vi "J1939 - Workspace Control.vi"() -> ()   [LabVIEW 2019, in "J1939 Workspace Object.lvlib"]
doc: "Sample numeric display item."
uses:
  J1939 Workspace Object.lvlib
  <vilib>/NI VeriStand/Display Template Support/DisplayTemplateSupport.llb/cluster_Screen Item Settings.ctl
  <vilib>/NI VeriStand/Display Template Support/DisplayTemplateSupport.llb/cluster_Graph Scale Settings.ctl
  <vilib>/NI VeriStand/Display Template Support/DisplayTemplateSupport.llb/cluster_Graph Plot Settings.ctl
  NationalInstruments.VeriStand.SystemStorage
  Workspace Shared/Types/UI.StateVariables.ctl
  <vilib>/NI VeriStand/Display Template Support/DisplayTemplateSupport.llb/enum_Display Template Handler Minimal To Widget Msg.ctl
  <vilib>/NI VeriStand/Execution/Workspace/SystemStateRegEventRef.ctl
  <vilib>/NI VeriStand/Execution/Workspace/Target State Info.ctl
  <vilib>/NI VeriStand/Execution/Workspace/Target State.ctl
  Shared/Types/Private Data.ctl
  <vilib>/NI/STM/TCP/TCP Connection Info.ctl
  <vilib>/NI/STM/SubVIs/MetaDataElement.ctl
  Shared/Types/Error Cluster.ctl
  Shared/Types/Error Types.ctl
  <vilib>/NI VeriStand/Display Template Support/DisplayTemplateSupport.llb/enum_Display Template Handler Minimal To Workspace.ctl
  <vilib>/NI VeriStand/Execution/Workspace/WorkspaceAPI.ctl
  <vilib>/NI VeriStand/Execution/Workspace/SystemStateEventRef.ctl
  Workspace Shared/Types/UI.Refs.ctl
  <vilib>/Utility/miscctls.llb/LVStringsAndValuesArrayTypeDef_U8.ctl
  Shared/J1939 Utilities/SubVIs/Convert CAN Arb ID to J1939 ID.vi
  <vilib>/NI VeriStand/Display Template Support/DisplayTemplateSupport.llb/sub_Display Template Handler Custom.vi
  Shared/J1939 Addon Shared.lvlib
  <vilib>/NI/STM/NI STM.lvlib
  Workspace Shared/J1939 Workspace Shared.lvlib
  <vilib>/NI VeriStand/Execution/Workspace/NI_VS Workspace ExecutionAPI.lvlib
  Shared/J1939 Utilities/J1939 Utilities.lvlib
  NationalInstruments.VeriStand.ClientAPI
panel:
  in  "Tab Control":enum32{"DTCs", "Custom RQST", "RAW FRAME"}(tab)
  in  "Refresh Continuous":bool
  in  "Clear DTC":bool
  in  "Refresh DTCs":bool
  in  "DTCs":i32(listbox)
  in  "Addresses":string(tree)
  in  "Refresh Addresses":bool
  out "Response":string
  in  "Request":bool
  in  "PGN":u32 format="%.0x"
  in  "DA":u8(ring)
  in  "Clear Array":bool
  in  "RAW":bool
  out "Priority":u8 format="%02x"
  out "SA":u8 format="%02x"
  out "PGN":u32 format="%06x"
  in  "Identifier":u32 format="%08x"
  in  "Data":u8[](array[numeric])=[0, 0, 0, 0, 0, 0, 0, 0] format="%.0x"
  in  "Errors":bool
  out "Device":string
  in  "NIVS.Workspace Event":refnum<event-registration>
  in  "NIVS.Gateway IP Address":string
  in  "NIVS.System Definition Root":refnum<k24>
  in  "Item.Data":T1
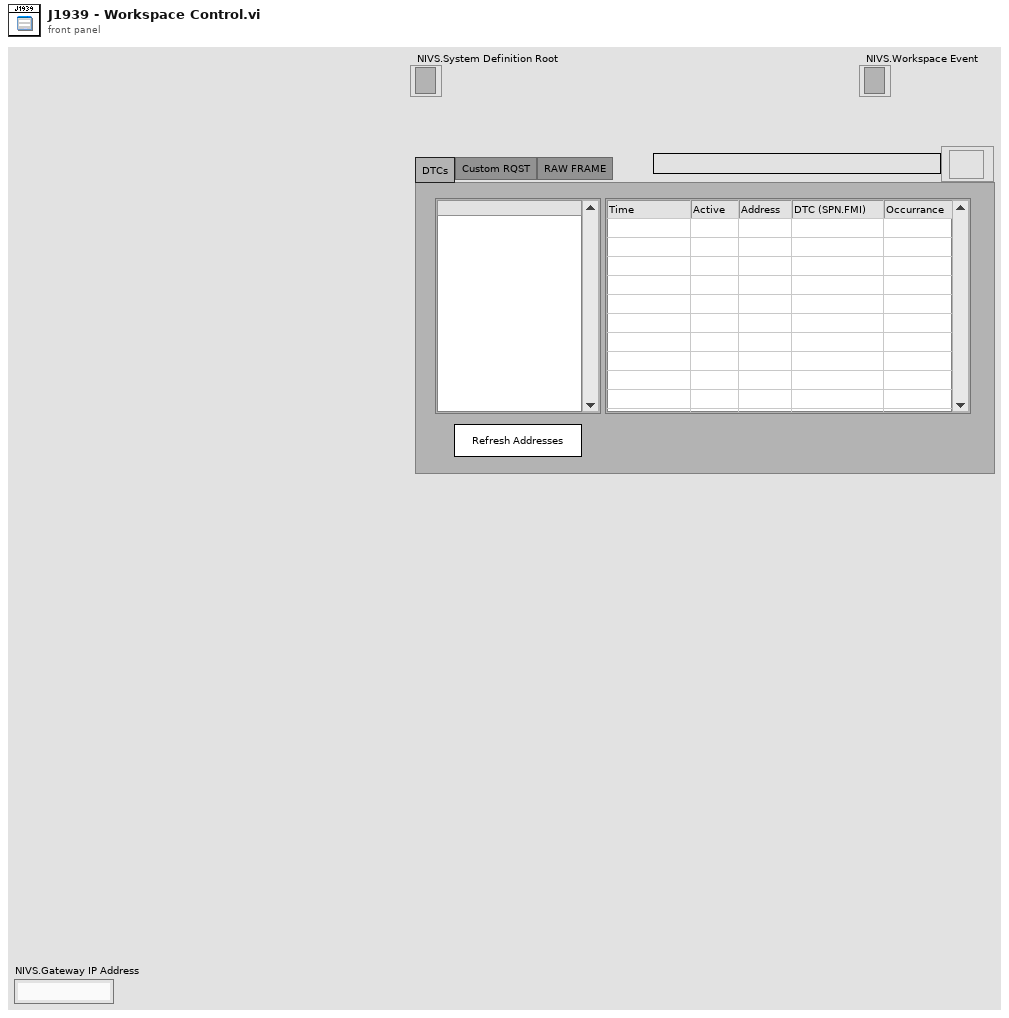
[diagram p1: front panel]
types:
  T1 = typedef "cluster_Screen Item Settings.ctl" = cluster{"Template VI":string, "Position X":i32, "Position Y":i32, "Custom":string, "Show Title Bar":bool, "ID":i32, "Always On Top":bool, "Allow Resize":bool, "Allow Minimize":bool, "Allow Close":bool, "Size to Screen":bool, "Screen.ID":i32, "State":enum16{"Normal", "New"}, "Title":string, "Window Bounds":cluster{"[0]":i16, "[1]":i16, "[2]":i16, "[3]":i16}, "Channel Ref":u64, "Unit":string, "Default Units?":bool, "Flash Limit?":bool, "Color 1":u32, "Color 2":u32, "Color 3":u32, "Color 4":u32, "Bck Color":u32, "Fore Color":u32, "Limit 1":dbl, "Limit 2":dbl, "Limit 3":dbl, "Limit 4":dbl, "Limit Mode 1":i32, "Limit Mode 2":i32, "Limit Mode 3":i32, "Limit Mode 4":i32, "Scale Precision":i32, "Scale Min":dbl, "Scale Max":dbl, "Format":i32, "Precision":i32, "Background Type":i32, "IDs":i32[], "Units":string[], "Labels":string[], "Scale Factor":dbl, "Scale Offset":dbl, "YScale Index":u32[], "XScale":T2, "YScales":T2[], "Plots":T3[], "Update Period":dbl, "History Length":dbl, "My.Ref":refnum<vi>, "Is Control?":bool, "Channel Paths":string[], "Custom Data":variant}
  T2 = typedef "cluster_Graph Scale Settings.ctl" = cluster{"Format":u8, "Precision":u8, "Fit":u8, "Label":string, "Use Default Label":bool, "Label Visible":bool, "Min":dbl, "Max":dbl}
  T3 = typedef "cluster_Graph Plot Settings.ctl" = cluster{"Bar Style":u8, "Fill To":i16, "Fill/PtColor":u32, "Line Style":u8, "Line Width":u8, "Color":u32, "Interp":u8, "Point Style":u8}
  T4 = typedef "J1939 Workspace Shared.lvlib/UI.StateVariables.ctl" = cluster{"NIVS.Gateway IP Address":string, "LaunchConfig.Ref":refnum<user-event>, "Events.Refs":cluster{"LaunchConfig":refnum<event-registration>, "SystemChange":T5, "NIVS.Workspace":refnum<event-registration>}, "State":T6, "TCP.Refs":T7, "Addresses.LUT":variant, "Errors.Q":refnum<queue>, "NIVS.SysDefRoot":refnum<k24>, "State.Notifier":refnum<user-event>, "NIVS.Workspace":T9, "DTCs.Refresh":bool, "NIVS.State.Refs":T10, "UI.Refs":T11, "Addon.Connected":bool, "DTCs.Timer":u32, "Mode.Tool?":bool}
  T5 = typedef "NI_VS Workspace ExecutionAPI.lvlib/SystemStateRegEventRef.ctl" = refnum<event-registration>
  T6 = typedef "J1939 Addon Shared.lvlib/Private Data.ctl" = cluster{"PGN":u32, "DA":u8, "CD Path":string, "CD IP":string}
  T7 = typedef "NI STM.lvlib/TCP Connection Info.ctl" = cluster{"connection ID":refnum<k5>, "meta data":T8[]}
  T8 = typedef "NI STM.lvlib/MetaDataElement.ctl" = string
  T9 = typedef "NI_VS Workspace ExecutionAPI.lvlib/WorkspaceAPI.ctl" = refnum<k24>
  T10 = typedef "NI_VS Workspace ExecutionAPI.lvlib/SystemStateEventRef.ctl" = cluster{"CustDatRef":refnum<user-event>, "EvtRef":refnum<k27>, "Target State User Event":refnum<user-event>}
  T11 = typedef "J1939 Workspace Shared.lvlib/UI.Refs.ctl" = cluster{"ParentVI":refnum<vi>, "DTCs":refnum<vi>, "Addresses":refnum<vi>, "Device":refnum<vi>, "Data":refnum<vi>, "Identifier":refnum<vi>, "PGN":refnum<vi>, "DA":refnum<vi>, "Refresh Continuous":refnum<vi>, "Errors":refnum<vi>, "Refresh Addresses":refnum<vi>, "Refresh DTCs":refnum<vi>, "Clear DTC":refnum<vi>, "Request":refnum<vi>, "Clear Array":refnum<vi>, "RAW":refnum<vi>, "SA":refnum<vi>, "PGN Ind":refnum<vi>, "Priority":refnum<vi>, "Response":refnum<vi>}
  T12 = typedef "enum_Display Template Handler Minimal To Workspace.ctl" = cluster{"Operation":enum16{"SetCustomData", "DeleteItem"}, "Data":variant}
  T13 = typedef "enum_Display Template Handler Minimal To Widget Msg.ctl" = enum16{"Stop", "LaunchConfigDialog"}
  T14 = enum8{"Enabled", "Disabled", "Disabled and Grayed Out"}
  T15 = typedef "LVStringsAndValuesArrayTypeDef_U8.ctl" = cluster{"String":string, "Value":u8}[]
  T16 = cluster{"LaunchConfig":refnum<event-registration>, "SystemChange":T5, "NIVS.Workspace":refnum<event-registration>}
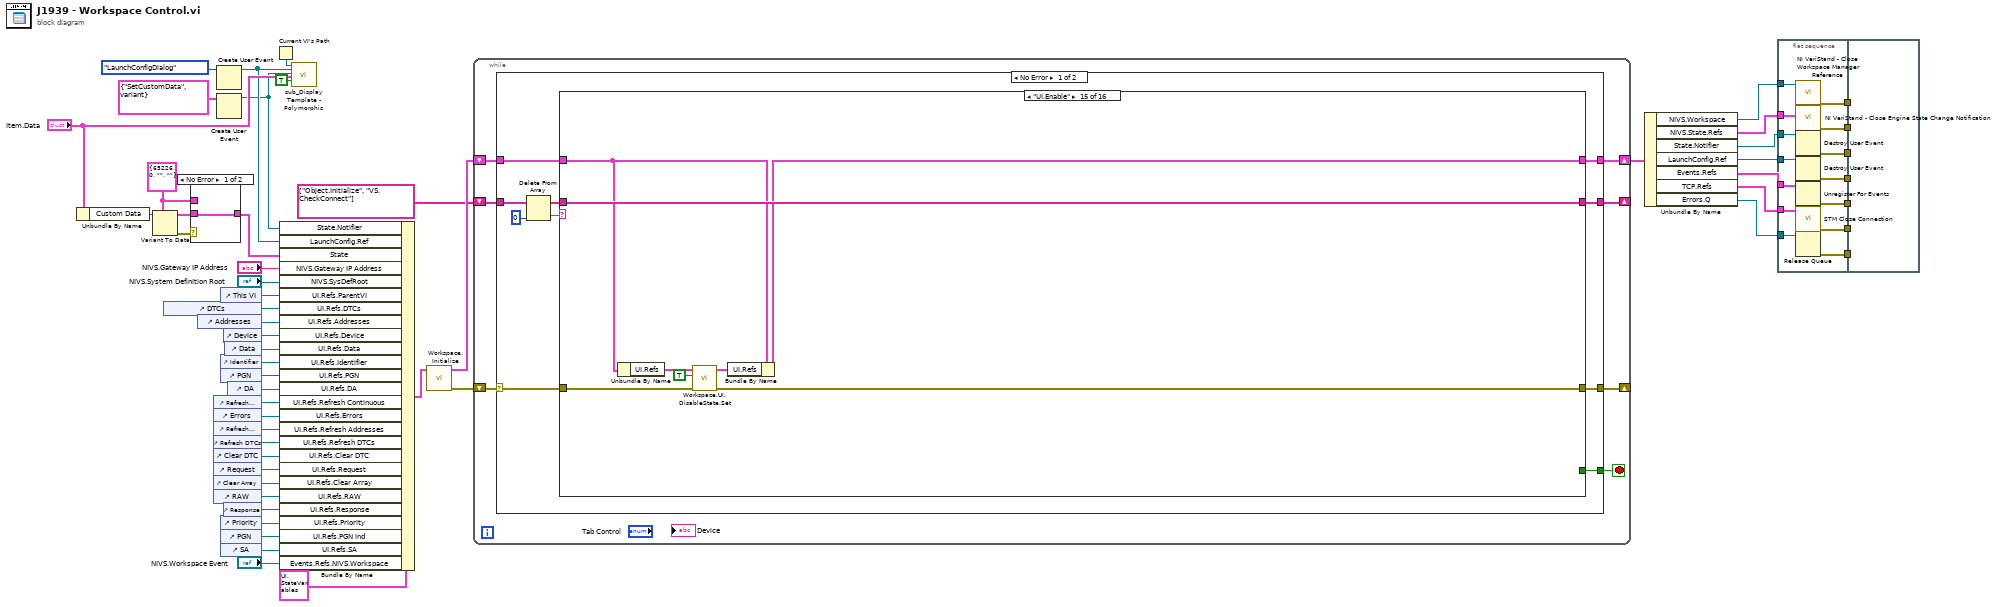
[diagram p0: block diagram]
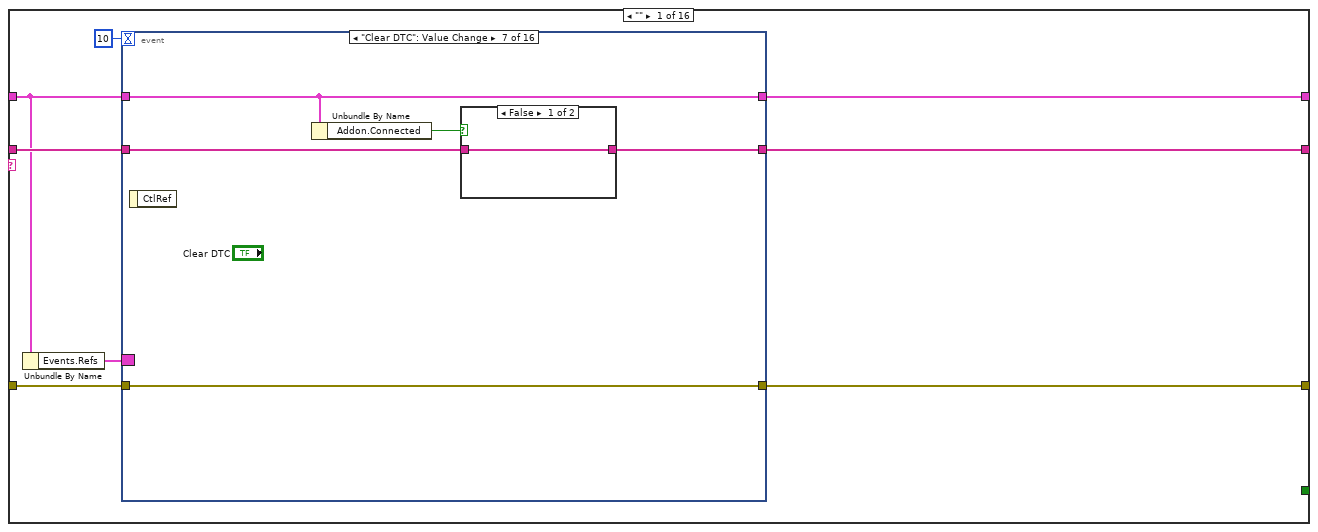
[diagram p2: hidden frame]
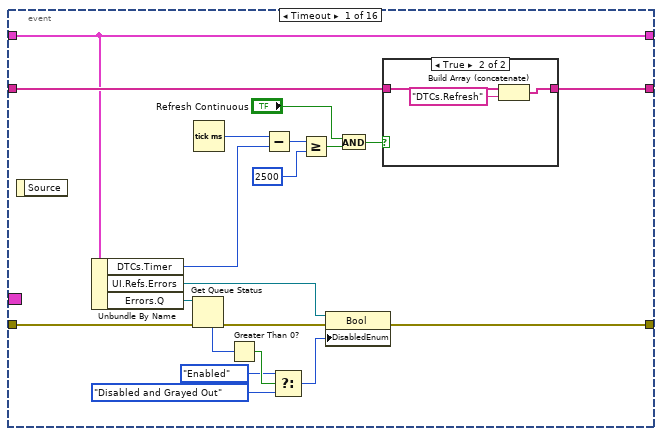
[diagram p3: hidden frame]
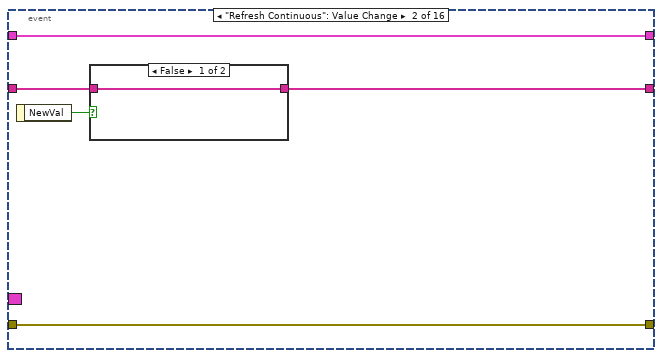
[diagram p5: hidden frame]
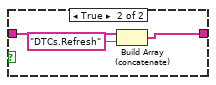
[diagram p6: hidden frame]
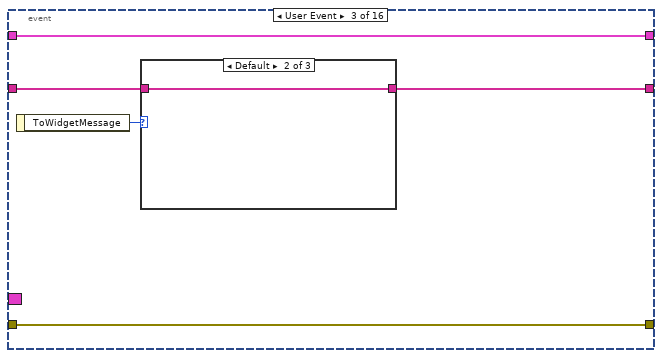
[diagram p7: hidden frame]
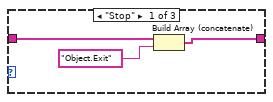
[diagram p8: hidden frame]
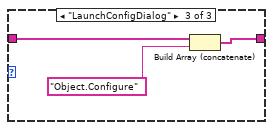
[diagram p9: hidden frame]
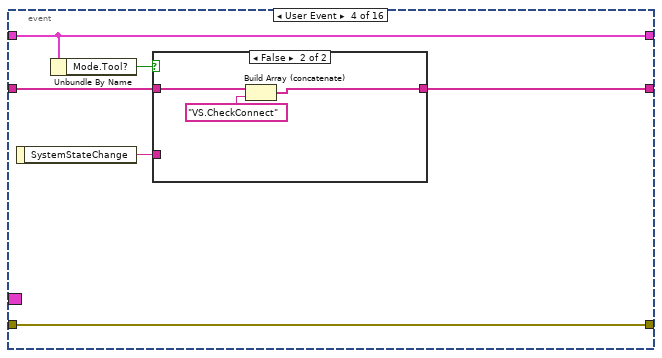
[diagram p10: hidden frame]
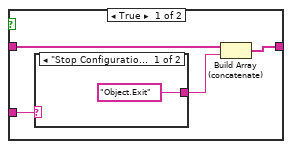
[diagram p11: hidden frame]
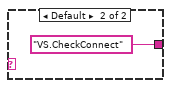
[diagram p12: hidden frame]
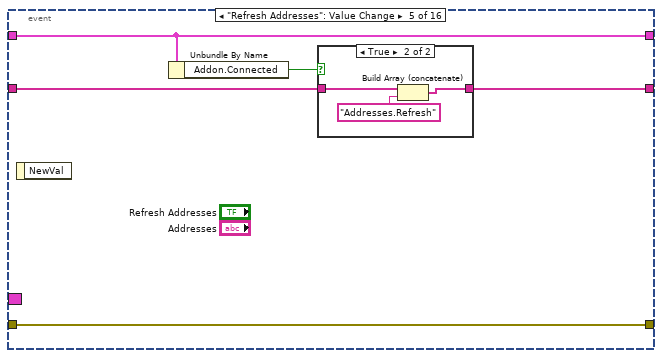
[diagram p13: hidden frame]
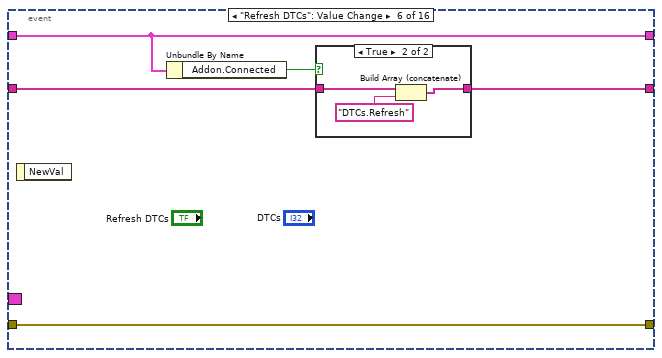
[diagram p15: hidden frame]
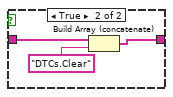
[diagram p17: hidden frame]
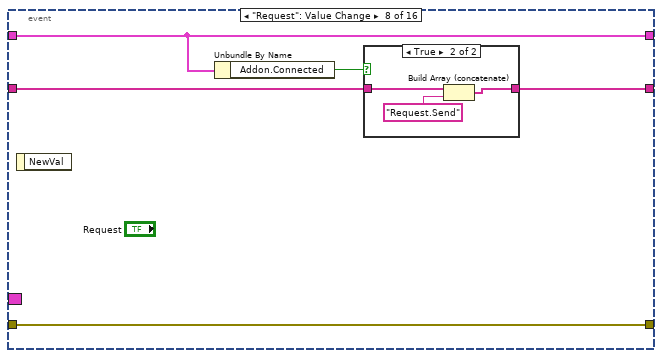
[diagram p18: hidden frame]
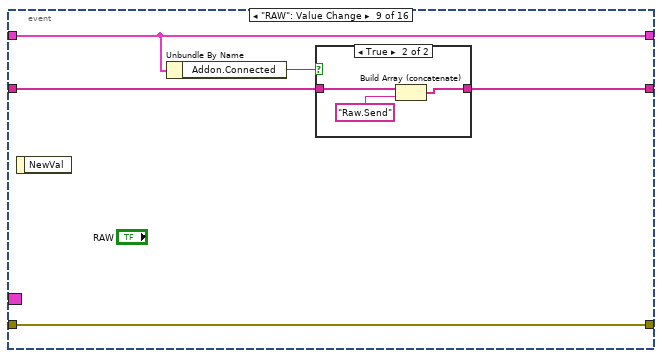
[diagram p20: hidden frame]
diagram:
  w51 = T6 {"PGN"=65226, "DA"=0, "CD Path"="", "CD IP"=""} ("Cluster")
  n1 = Unbundle By Name("Item.Data") -> ("Custom Data"=w48:variant)
  n2 = Variant To Data(type=w51, Variant=w48) -> (data=w50:T6, error out=w49:errorcluster)  [unwired: 1 in]
  n3 = control-ref of="DTCs"() -> (w35:refnum<vi>)
  n4 = case shown="No Error" w49 {
    tunnel: w50 -> [w56 _]
    tunnel: [w56 w57] -> w7
    tunnel: w51 -> [_ w57]
    frame No Error {
    }
    frame Error {
    }
  }
  n5 = control-ref of="Addresses"() -> (w34:refnum<vi>)
  n6 = control-ref of="Refresh Continuous"() -> (w28:refnum<vi>)
  n7 = control-ref of="Errors"() -> (w27:refnum<vi>)
  n8 = control-ref of="Refresh Addresses"() -> (w26:refnum<vi>)
  n9 = control-ref of="Refresh DTCs"() -> (w25:refnum<vi>)
  n10 = control-ref of="Clear DTC"() -> (w24:refnum<vi>)
  n11 = control-ref of="Request"() -> (w23:refnum<vi>)
  n12 = control-ref of="Clear Array"() -> (w22:refnum<vi>)
  n13 = control-ref of="RAW"() -> (w21:refnum<vi>)
  n14 = Create User Event(user event datatype=enum_Display_Template_Handler_Minimal_To_Widget_Msg."LaunchConfigDialog" ("ToWidgetMessage")) -> (user event=w6:refnum<user-event>)  [unwired: 1 in, 1 out]
  n15 = Create User Event(user event datatype=T12 {"Operation"=enum."SetCustomData", "Data"=variant} ("Data")) -> (user event=w5:refnum<user-event>)  [unwired: 1 in, 1 out]
  n16 = control-ref of="This VI"() -> (w36:refnum<vi>)
  n17 = control-ref of="Identifier"() -> (w31:refnum<vi>)
  n18 = control-ref of="PGN"() -> (w30:refnum<vi>)
  n19 = control-ref of="Priority"() -> (w2:refnum<vi>)
  n20 = control-ref of="PGN"() -> (w3:refnum<vi>)
  n21 = control-ref of="SA"() -> (w4:refnum<vi>)
  n22 = control-ref of="Device"() -> (w33:refnum<vi>)
  n23 = control-ref of="Response"() -> (w1:refnum<vi>)
  n24 = control-ref of="Data"() -> (w32:refnum<vi>)
  n25 = control-ref of="DA"() -> (w29:refnum<vi>)
  n26 = Current VI's Path() -> (path=w53:path)
  n27 = Bundle By Name(cluster=T4 {"NIVS.Gateway IP Address"="", "LaunchConfig.Ref"=refnum, "Events.Refs"={"LaunchConfig"=refnum, "SystemChange"=refnum, "NIVS.Workspace"=refnum}, "State"={"PGN"=0, "DA"=0, "CD Path"="", "CD IP"=""}, "TCP.Refs"={"connection ID"=refnum, "meta data"=[]}, "Addresses.LUT"=variant, "Errors.Q"=refnum, "NIVS.SysDefRoot"=refnum, "State.Notifier"=refnum, "NIVS.Workspace"=refnum, "DTCs.Refresh"=FALSE, "NIVS.State.Refs"={"CustDatRef"=refnum, "EvtRef"=refnum, "Target State User Event"=refnum}, "UI.Refs"={"ParentVI"=refnum, "DTCs"=refnum, "Addresses"=refnum, "Device"=refnum, "Data"=refnum, "Identifier"=refnum, "PGN"=refnum, "DA"=refnum, "Refresh Continuous"=refnum, "Errors"=refnum, "Refresh Addresses"=refnum, "Refresh DTCs"=refnum, "Clear DTC"=refnum, "Request"=refnum, "Clear Array"=refnum, "RAW"=refnum, "SA"=refnum, "PGN Ind"=refnum, "Priority"=refnum, "Response"=refnum}, "Addon.Connected"=FALSE, "DTCs.Timer"=0, "Mode.Tool?"=FALSE}, "State.Notifier"=w5, "LaunchConfig.Ref"=w6, "State"=w7, "NIVS.Gateway IP Address"="NIVS.Gateway IP Address", "NIVS.SysDefRoot"="NIVS.System Definition Root", "UI.Refs.ParentVI"=w36, "UI.Refs.DTCs"=w35, "UI.Refs.Addresses"=w34, "UI.Refs.Device"=w33, "UI.Refs.Data"=w32, "UI.Refs.Identifier"=w31, "UI.Refs.PGN"=w30, "UI.Refs.DA"=w29, "UI.Refs.Refresh Continuous"=w28, "UI.Refs.Errors"=w27, "UI.Refs.Refresh Addresses"=w26, "UI.Refs.Refresh DTCs"=w25, "UI.Refs.Clear DTC"=w24, "UI.Refs.Request"=w23, "UI.Refs.Clear Array"=w22, "UI.Refs.RAW"=w21, "UI.Refs.Response"=w1, "UI.Refs.Priority"=w2, "UI.Refs.PGN Ind"=w3, "UI.Refs.SA"=w4, "Events.Refs.NIVS.Workspace"="NIVS.Workspace Event") -> (w38:T4)
  n28 = call-poly <vilib>:"sub_Display Template - Polymorphic.vi"("Parent.Path"=w53, "ToWidgetEvent"=w6, "ToWorkspace"=w5, "Item.Data"="Item.Data", "Resizable"=TRUE) -> ()  [unwired: 1 in, 14 out]
  n29 = call "Workspace.Initialize.vi"("State"=w38) -> ("error out"=w37:errorcluster, "State"=w20:T4)  [unwired: 9 in]
  n30 = while {
    shift-right: [w62] -> _
    shift-left: w37 -> [w63]
    shift-right: [w58] -> w18
    shift-left: w20 -> [w61]
    shift-right: [w59] -> _
    shift-left: string[] ["Object.Initialize", "VS.CheckConnect"] -> [w60]
    stop <- w64 stop-if-true
    n31 = case shown="No Error" w63 {
      selector: w63 -> [w65 w473]
      tunnel: [w74 FALSE] -> w64
      tunnel: [w66 w471] -> w62
      tunnel: w61 -> [w73 w468]
      tunnel: w60 -> [w71 w469]
      tunnel: [w68 w469] -> w59
      tunnel: [w67 w468] -> w58
      frame No Error {
        n32 = Delete From Array(array=w71, index=0) -> (deleted portion=w70:string, array with subset deleted=w69:string[])  [unwired: 1 in]
        n33 = case shown="\"UI.Enable\"" w70 {
          selector: w70 -> [_ _ _ _ _ _ _ _ _ _ _ _ _ _ _ w463]
          tunnel: [_ _ _ _ _ _ _ _ TRUE _ _ _ _ _ _ _] -> w74
          tunnel: w73 -> [w76 w239 w248 w265 w318 w323 w357 w385 w388 w393 w417 w425 w437 w449 w454 w466]
          tunnel: w69 -> [w80 w246 w258 w274 w319 w321 w363 w381 w389 w391 w418 w426 w433 w451 w461 w467]
          tunnel: [w81 w246 w258 w274 w319 w320 w362 w381 w389 w390 w418 w426 w433 w451 w461 w467] -> w68
          tunnel: [w79 w236 w247 w275 w318 w322 w356 w384 w388 w394 w417 w424 w434 w450 w455 w466] -> w67
          tunnel: [w78 w235 w257 w260 w295 w326 w359 w380 w387 w402 w413 w419 w432 w452 w456 w465] -> w66
          tunnel: w65 -> [w77 w235 w257 w261 w292 w327 w358 w380 w387 w403 w412 w419 w432 w453 w457 w465]
          frame "" {
            n34 = Unbundle By Name(w76) -> ("Events.Refs"=w75:T16)
            n35 = event shown="[6] \"Clear DTC\": Value Change" {
              selector: w75 -> [_ _ _ _ _ _ _ _ _ _ _ _ _ _ _ _]
              dyn-events: _ -> [_ _ _ _ _ _ _ _ _ _ _ _ _ _ _ _]
              timeout: 10 -> [_ _ _ _ _ _ _ _ _ _ _ _ _ _ _ _]
              tunnel: w76 -> [w91 w110 w120 w129 w146 w154 w161 w172 w181 w190 w199 w203 w210 w220 w225 w234]
              tunnel: [w92 w108 w116 w132 w144 w152 w162 w170 w179 w188 w198 w204 w212 w216 w222 w231] -> w81
              tunnel: w80 -> [w93 w109 w117 w133 w145 w153 w163 w171 w180 w189 w201 w204 w212 w217 w223 w232]
              tunnel: [w91 w110 w120 w129 w146 w154 w161 w172 w181 w190 w199 w203 w210 w220 w225 w234] -> w79
              tunnel: [w85 w111 w119 w130 w147 w156 w165 w174 w183 w192 w200 w202 w211 w219 w224 w233] -> w78
              tunnel: w77 -> [w87 w111 w119 w130 w147 w156 w165 w174 w183 w192 w200 w202 w211 w219 w224 w233]
              event Timeout {
                n36 = event-data() -> ()  [unwired: 2 out]
                n37 = Unbundle By Name(w91) -> ("DTCs.Timer"=w84:u32, "UI.Refs.Errors"=w89:refnum<vi>, "Errors.Q"=w90:refnum<queue>)
                n38 = Get Queue Status(queue=w90, error in (no error)=w87) -> (error out=w88:errorcluster, # elements in queue=w102:i32)  [unwired: 1 in, 6 out]
                n39 = Tick Count (ms)() -> (millisecond timer value=w96:u32)
                n40 = Greater Than 0?(x=w102) -> (x > 0?=w101:bool)
                n41 = Subtract(x=w96, y=w84) -> (x-y=w98:u32)
                n42 = Select(t=T14."Enabled" ("Disabled"), s=w101, f=T14."Disabled and Grayed Out") -> (s? t:f=w86:T14)
                n43 = Greater Or Equal?(x=w98, y=u32 2500) -> (x >= y?=w83:bool)
                n44 = property class="Bool"(reference=w89, error in=w88, "DisabledEnum"=w86) -> (error out=w85:errorcluster)  [unwired: 1 out]
                n45 = And(x="Refresh Continuous", y=w83) -> (x .and. y?=w94:bool)
                n46 = case shown="True" w94 {
                  tunnel: w93 -> [w103 w105]
                  tunnel: [w103 w104] -> w92
                  frame False {
                  }
                  frame True {
                    n47 = Build Array (concatenate)(w105, "DTCs.Refresh" ("NewVal")) -> (w104:string[])
                  }
                }
              }
              event "Refresh Continuous": Value Change {
                n48 = event-data() -> ("NewVal"=w107:bool)  [unwired: 1 out]
                n49 = case shown="False" w107 {
                  tunnel: w109 -> [w112 w114]
                  tunnel: [w112 w113] -> w108
                  frame False {
                  }
                  frame True {
                    n50 = Build Array (concatenate)(w114, "DTCs.Refresh" ("NewVal")) -> (w113:string[])
                  }
                }
              }
              event User Event {
                n51 = event-data() -> ("ToWidgetMessage"=w118:T13)  [unwired: 1 out]
                n52 = case shown="Default" w118 {
                  tunnel: w117 -> [w123 w124 w127]
                  tunnel: [w122 w124 w126] -> w116
                  frame "Stop" {
                    n53 = Build Array (concatenate)(w123, "Object.Exit") -> (w122:string[])
                  }
                  frame Default {
                  }
                  frame "LaunchConfigDialog" {
                    n54 = Build Array (concatenate)(w127, "Object.Configure") -> (w126:string[])
                  }
                }
              }
              event User Event {
                n55 = event-data() -> ("SystemStateChange"=w128:string)  [unwired: 1 out]
                n56 = Unbundle By Name(w129) -> ("Mode.Tool?"=w131:bool)
                n57 = case shown="False" w131 {
                  tunnel: w133 -> [w137 w142]
                  tunnel: [w136 w141] -> w132
                  tunnel: w128 -> [w135 _]
                  frame True {
                    # "System state not connected"
                    n58 = case shown="\"Stop Configuration\"" w135 {
                      tunnel: ["Object.Exit" "VS.CheckConnect"] -> w134
                      frame "Stop Configuration" {
                      }
                      frame Default {
                      }
                    }
                    n59 = Build Array (concatenate)(w137, w134) -> (w136:string[])
                  }
                  frame False {
                    # "System state is connected"
                    n60 = Build Array (concatenate)(w142, "VS.CheckConnect") -> (w141:string[])
                  }
                }
              }
              event "Refresh Addresses": Value Change {
                n61 = event-data() -> ()  [unwired: 2 out]
                n62 = Unbundle By Name(w146) -> ("Addon.Connected"=w143:bool)
                n63 = case shown="True" w143 {
                  tunnel: w145 -> [w148 w150]
                  tunnel: [w148 w149] -> w144
                  frame False {
                  }
                  frame True {
                    n64 = Build Array (concatenate)(w150, "Addresses.Refresh") -> (w149:string[])
                  }
                }
              }
              event "Refresh DTCs": Value Change {
                n65 = event-data() -> ()  [unwired: 2 out]
                n66 = Unbundle By Name(w154) -> ("Addon.Connected"=w155:bool)
                n67 = case shown="True" w155 {
                  tunnel: w153 -> [w157 w159]
                  tunnel: [w157 w158] -> w152
                  frame False {
                  }
                  frame True {
                    n68 = Build Array (concatenate)(w159, "DTCs.Refresh") -> (w158:string[])
                  }
                }
              }
              event "Clear DTC": Value Change {
                n69 = event-data() -> ()  [unwired: 2 out]
                n70 = Unbundle By Name(w161) -> ("Addon.Connected"=w164:bool)
                n71 = case shown="False" w164 {
                  tunnel: w163 -> [w166 w168]
                  tunnel: [w166 w167] -> w162
                  frame False {
                  }
                  frame True {
                    n72 = Build Array (concatenate)(w168, "DTCs.Clear") -> (w167:string[])
                  }
                }
              }
              event "Request": Value Change {
                n73 = event-data() -> ()  [unwired: 2 out]
                n74 = Unbundle By Name(w172) -> ("Addon.Connected"=w173:bool)
                n75 = case shown="True" w173 {
                  tunnel: w171 -> [w175 w177]
                  tunnel: [w175 w176] -> w170
                  frame False {
                  }
                  frame True {
                    n76 = Build Array (concatenate)(w177, "Request.Send") -> (w176:string[])
                  }
                }
              }
              event "RAW": Value Change {
                n77 = event-data() -> ()  [unwired: 2 out]
                n78 = Unbundle By Name(w181) -> ("Addon.Connected"=w182:bool)
                n79 = case shown="True" w182 {
                  tunnel: w180 -> [w184 w186]
                  tunnel: [w184 w185] -> w179
                  frame False {
                  }
                  frame True {
                    n80 = Build Array (concatenate)(w186, "Raw.Send") -> (w185:string[])
                  }
                }
              }
              event "Clear Array": Value Change {
                n81 = event-data() -> ()  [unwired: 2 out]
                n82 = Unbundle By Name(w190) -> ("Addon.Connected"=w191:bool)
                n83 = case shown="True" w191 {
                  tunnel: w189 -> [w193 w195]
                  tunnel: [w193 w194] -> w188
                  frame False {
                  }
                  frame True {
                    n84 = Build Array (concatenate)(w195, "Raw.Clear") -> (w194:string[])
                  }
                }
              }
              event "Addresses": Value Change {
                n85 = event-data() -> ()  [unwired: 2 out]
                n86 = Build Array (concatenate)(w201, "DTCs.Refresh" ("NewVal")) -> (w198:string[])
              }
              event "Identifier": Value Change {
                n87 = event-data() -> ("NewVal"=w205:u32)  [unwired: 1 out]
                n88 = call-poly "Common Conversions.vi"("Arb ID"=w205) -> ("Priority"=→"Priority":u8, "PGN"=→"PGN":u32, "Source Address"=→"SA":u8)  [unwired: 11 in, 1 out]
              }
              event "Errors": Value Change {
                n89 = event-data() -> ()  [unwired: 2 out]
                n90 = Unbundle By Name(w210) -> ("Errors.Q"=w209:refnum<queue>)
                n91 = flat-sequence {
                  tunnel: [w214] -> w213
                  tunnel: w209 -> [w214]
                  frame #0 {
                  }
                }
                n92 = call "Error Display.vi"("queue out"=w213) -> ()  [unwired: 11 in]
              }
              event Panel Close? {
                n93 = event-data() -> ()  [unwired: 5 out]
                n94 = Build Array (concatenate)(w217, "Object.Exit") -> (w216:string[])
                n95 = event-data("Discard?"=TRUE) -> ()  [unwired: 1 in, 1 out]
              }
              event User Event {
                n96 = event-data() -> ("Workspace Event"=w221:string)  [unwired: 1 out]
                n97 = case shown="\"Disconnect\", \"Shut Down\"" w221 {
                  tunnel: w223 -> [w226 w229]
                  tunnel: [w226 w228] -> w222
                  frame Default {
                  }
                  frame "Disconnect", "Shut Down" {
                    n98 = Build Array (concatenate)(w229, "Object.Exit") -> (w228:string[])
                  }
                }
              }
              event Menu Selection (User) {
                n99 = event-data() -> ("ItemTag"=w230:string)  [unwired: 1 out]
                n100 = Build Array (concatenate)(w232, w230) -> (w231:string[])
              }
            }
          }
          frame "Addresses.Refresh" {
            n101 = Unbundle By Name(w239) -> ("UI.Refs.Addresses"=w245:refnum<vi>, "UI.Refs.DA"=w244:refnum<vi>, "TCP.Refs"=w243:T7, "State"=w242:T6, "Errors.Q"=w241:refnum<queue>, "UI.Refs.ParentVI"=w240:refnum<vi>)
            n102 = call "Request Addresses Event.vi"("connection info"=w243, "DA"=w244, "Addresses"=w245, "State Variables"=w242, "Error Q"=w241, "VI Ref"=w240) -> ("connection info"=w238:T7, "Address Lookup Table Out"=w237:variant)  [unwired: 8 in]
            n103 = Bundle By Name(cluster=w239, "TCP.Refs"=w238, "Addresses.LUT"=w237) -> (w236:T4)
          }
          frame "DTCs.Clear" {
            n104 = Unbundle By Name(w248) -> ("UI.Refs.Addresses"=w251:refnum<vi>, "TCP.Refs"=w256:T7, "State"=w255:T6, "Addresses.LUT"=w254:variant, "Errors.Q"=w253:refnum<queue>, "UI.Refs.ParentVI"=w252:refnum<vi>)
            n105 = call "Clear DTCs Event.vi"("connection info"=w256, "Addresses"=w251, "State Variables"=w255, "Address Lookup Table"=w254, "Error Q"=w253, "VI Ref"=w252) -> ("connection info"=w250:T7, "Address Lookup Table Out"=w249:variant)  [unwired: 8 in]
            n106 = Bundle By Name(cluster=w248, "TCP.Refs"=w250, "Addresses.LUT"=w249) -> (w247:T4)
          }
          frame "DTCs.Refresh" {
            n107 = Unbundle By Name(w265) -> ("UI.Refs.DTCs"=w272:refnum<vi>, "UI.Refs.Addresses"=w271:refnum<vi>, "TCP.Refs"=w270:T7, "State"=w269:T6, "Addresses.LUT"=w268:variant, "Errors.Q"=w267:refnum<queue>, "UI.Refs.ParentVI"=w266:refnum<vi>, "UI.Refs.Refresh Continuous"=w262:refnum<vi>)
            n108 = property class="Bool (strict)"(reference=w262, error in=w261) -> (error out=w260:errorcluster, "Value"=w259:bool)  [unwired: 1 out]
            n109 = Not(x=w259) -> (.not. x?=w273:bool)
            n110 = flat-sequence {
              tunnel: w268 -> [w288]
              tunnel: w270 -> [w286]
              tunnel: w269 -> [w284]
              tunnel: w273 -> [w283]
              tunnel: [w287] -> w278
              tunnel: [w285] -> w277
              tunnel: w272 -> [w282]
              tunnel: w271 -> [w281]
              tunnel: w267 -> [w280]
              tunnel: w266 -> [w279]
              tunnel: [w290] -> w263
              tunnel: [w291] -> w264
              tunnel: w278 -> [w291]
              tunnel: w277 -> [w290]
              tunnel: [w289] -> w276
              frame #0 {
                n111 = call "Refresh DTCs Event.vi"("connection info"=w286, "Addresses"=w281, "DTCs"=w282, "State Variables"=w284, "Address Lookup Table"=w288, "To Top (T)"=w283, "Error Q"=w280, "VI Ref"=w279) -> ("connection info"=w285:T7, "Address Lookup Table Out"=w287:variant)  [unwired: 6 in]
              }
              frame #1 {
                n112 = Tick Count (ms)() -> (millisecond timer value=w289:u32)
              }
            }
            n113 = Bundle By Name(cluster=w265, "DTCs.Timer"=w276, "TCP.Refs"=w263, "Addresses.LUT"=w264) -> (w275:T4)
          }
          frame "Object.Initialize" {
            n114 = Unbundle By Name(w318) -> ("UI.Refs.Errors"=w293:refnum<vi>, "UI.Refs.Data"=w300:refnum<vi>, "UI.Refs.Identifier"=w304:refnum<vi>, "UI.Refs.DA"=w306:refnum<vi>, "UI.Refs.PGN"=w309:refnum<vi>, "UI.Refs.DTCs"=w312:refnum<vi>, "UI.Refs.Addresses"=w315:refnum<vi>, "UI.Refs.Refresh Continuous"=w316:refnum<vi>)
            n115 = property class="Bool (strict)"(reference=w316, error in=w292, "Value"=FALSE) -> (error out=w313:errorcluster)  [unwired: 1 out]
            n116 = invoke class="Tree (strict)" method="Edit Tree Items.Delete"(reference=w315, error in=w313, "Delete Children"=TRUE ("Delete Children?")) -> (error out=w310:errorcluster)  [unwired: 2 in, 4 out]
            n117 = property class="MCListbox (strict)"(reference=w312, error in=w310, "ItemNames"=string[][] [] ("Item Names")) -> (error out=w307:errorcluster)  [unwired: 1 out]
            n118 = property class="DigNum (strict)"(reference=w309, error in=w307, "Value"=u32 0) -> (error out=w305:errorcluster)  [unwired: 1 out]
            n119 = property class="Ring (strict)"(reference=w306, error in=w305, "Value"=u8 0, "StringsAndValues[]"=T15 [] ("Strings And Values []")) -> (error out=w303:errorcluster)  [unwired: 1 out]
            n120 = property class="DigNum (strict)"(reference=w304, error in=w303, "Val(Sgnl)"=u32 0 ("Value (Signaling)")) -> (error out=w299:errorcluster)  [unwired: 1 out]
            n121 = property class="Arr (strict)"(reference=w300, error in=w299, "Value"=u8[] []) -> (error out=w296:errorcluster)  [unwired: 1 out]
            n122 = property class="Bool"(reference=w293, error in=w296, "DisabledEnum"=T14."Disabled and Grayed Out" ("f")) -> (error out=w295:errorcluster)  [unwired: 1 out]
          }
          frame "Object.Configure" {
            n123 = Unbundle By Name(w323) -> ("State"=w325:T6, "State.Notifier"=w328:refnum<user-event>, "NIVS.SysDefRoot"=w329:refnum<k24>, "State.CD Path"=w332:string)
            n124 = call "Select Custom Device.vi"("CD Path"=w332, "NIVS.System Definition Root"=w329) -> ("Cancelled?"=w330:bool, "IP Address"=w333:string, "Custom Device Path Out"=w331:string)  [unwired: 7 in]
            n125 = case shown="False" w330 {
              tunnel: w328 -> [w335 _]
              tunnel: w333 -> [w341 _]
              tunnel: w331 -> [w342 _]
              tunnel: w327 -> [w339 w353]
              tunnel: [w339 w353] -> w326
              tunnel: w325 -> [w340 w352]
              tunnel: [w334 w352] -> w324
              tunnel: w321 -> [w338 w351]
              tunnel: [w336 w351] -> w320
              frame False {
                n126 = flat-sequence {
                  tunnel: w342 -> [w350]
                  tunnel: w341 -> [w349]
                  tunnel: w340 -> [w348]
                  tunnel: w335 -> [w345]
                  tunnel: [w344] -> w334
                  tunnel: [w343] -> _
                  frame #0 {
                    n127 = Bundle By Name(cluster=w348, "CD Path"=w350, "CD IP"=w349) -> (w344:T6)
                    n128 = Bundle By Name(cluster=T12 {"Operation"=enum."SetCustomData", "Data"=variant} ("event data"), "Data"=w344) -> (w346:T12)
                    n129 = Generate User Event(user event=w345, event data cluster=w346) -> (error out=w343:errorcluster)  [unwired: 2 in, 1 out]
                  }
                }
                n130 = Build Array (concatenate)(w338, "VS.CheckConnect") -> (w336:string[])
              }
              frame True {
              }
            }
            n131 = Bundle By Name(cluster=w323, "State"=w324) -> (w322:T4)
          }
          frame "Object.Connected" {
            n132 = Unbundle By Name(w357) -> ("TCP.Refs"=w355:T7, "State.CD IP"=w360:string, "State.CD Path"=w361:string)
            n133 = call "STM Close Connection.vi"("connection info"=w355) -> ("error out"=w354:errorcluster)  [unwired: 10 in]
            n134 = flat-sequence {
              tunnel: w363 -> [w375]
              tunnel: [w373] -> w362
              tunnel: w361 -> [w365]
              tunnel: w360 -> [w372]
              tunnel: [w370] -> w359
              tunnel: w358 -> [w369]
              tunnel: w357 -> [w367]
              tunnel: [w366] -> w356
              tunnel: w354 -> [_]
              frame #0 {
                n135 = call "UI.Addon.Path.Parse.vi"("Cached Addon Path"=w365) -> ("Addon Name"=w364:string)  [unwired: 6 in, 4 out]
                n136 = call "Open Connection to Target.vi"("error in (no error)"=w369, "IP Address"=w372, "TCP Service"=w364) -> ("error out"=w371:errorcluster, "connection info"=w368:T7)  [unwired: 7 in]
                n137 = Bundle By Name(cluster=w367, "TCP.Refs"=w368) -> (w366:T4)
                n138 = case shown="No Error" w371 {
                  selector: w371 -> [w377 w379]
                  tunnel: [string[] ["Object.Initialize", "UI.Enable"] ("element") string[] ["Object.Initialize", "UI.Disable"] ("element")] -> w374
                  tunnel: [w377 w379] -> w370
                  frame No Error {
                  }
                  frame Error {
                  }
                }
                n139 = Build Array (concatenate)(w375, w374) -> (w373:string[])
              }
            }
          }
          frame "Object.Disconnected" {
            n140 = Unbundle By Name(w385) -> ("TCP.Refs"=w383:T7)
            n141 = Bundle By Name(cluster=w385, "TCP.Refs"=T7 {"connection ID"=refnum, "meta data"=[]}) -> (w384:T4)
            n142 = call "STM Close Connection.vi"("connection info"=w383) -> ()  [unwired: 10 in, 1 out]
          }
          frame "Object.Exit" {
          }
          frame "VS.CheckConnect" {
            n143 = Unbundle By Name(w393) -> ("UI.Refs.Device"=w400:refnum<vi>, "NIVS.Workspace"=w398:T9, "NIVS.SysDefRoot"=w399:refnum<k24>, "State.CD Path"=w397:string)
            n144 = Current VI's Menubar() -> (w401:refnum<k9>)
            n145 = call "UI.Connection.State.Get.vi"("Menu Ref"=w401, "Name Ref"=w400, "error in (no error)"=w403, "Addon Path in"=w397, "NIVS.System Definition Root in"=w399, "NIVS.Workspace Ref in"=w398) -> ("error out"=w402:errorcluster, "Addon Connected?"=w392:bool, "NIVS.System Definition Root out"=w395:refnum<k24>, "NIVS.Workspace Ref out"=w396:T9)  [unwired: 2 in]
            n146 = case shown="False" w392 {
              tunnel: w391 -> [w406 w409]
              tunnel: [w405 w408] -> w390
              frame False {
                n147 = Build Array (concatenate)(w406, string[] ["Object.Disconnected", "Object.Initialize", "UI.Disable"]) -> (w405:string[])
              }
              frame True {
                n148 = Build Array (concatenate)(w409, "Object.Connected") -> (w408:string[])
              }
            }
            n149 = Bundle By Name(cluster=w393, "NIVS.Workspace"=w396, "NIVS.SysDefRoot"=w395, "Addon.Connected"=w392) -> (w394:T4)
          }
          frame "Raw.Clear" {
            n150 = Unbundle By Name(w417) -> ("UI.Refs.Identifier"=w415:refnum<vi>, "UI.Refs.Data"=w416:refnum<vi>)
            n151 = property class="Arr (strict)"(reference=w416, error in=w412, "Value"=u8[] []) -> (error out=w414:errorcluster)  [unwired: 1 out]
            n152 = property class="DigNum (strict)"(reference=w415, error in=w414, "Val(Sgnl)"=u32 0 ("Value (Signaling)")) -> (error out=w413:errorcluster)  [unwired: 1 out]
          }
          frame "Raw.Send" {
            n153 = Unbundle By Name(w425) -> ("TCP.Refs"=w429:T7, "State"=w428:T6, "Addresses.LUT"=w427:variant, "Errors.Q"=w423:refnum<queue>, "UI.Refs.ParentVI"=w422:refnum<vi>)
            n154 = call "RAW Event.vi"("connection info"=w429, "State Variables"=w428, "Address Lookup Table"=w427, "Identifier"="Identifier", "Data"="Data", "Error Q"=w423, "VI Ref"=w422) -> ("connection info"=w421:T7, "Address Lookup Table Out"=w420:variant)  [unwired: 7 in]
            n155 = Bundle By Name(cluster=w425, "TCP.Refs"=w421, "Addresses.LUT"=w420) -> (w424:T4)
          }
          frame "Request.Send" {
            n156 = Unbundle By Name(w437) -> ("TCP.Refs"=w442:T7, "State"=w441:T6, "Addresses.LUT"=w440:variant, "Errors.Q"=w439:refnum<queue>, "UI.Refs.ParentVI"=w438:refnum<vi>)
            n157 = call "Request Event.vi"("connection info"=w442, "State Variables"=w441, "Address Lookup Table"=w440, "PGN"="PGN", "DA"="DA", "Error Q"=w439, "VI Ref"=w438) -> ("connection info"=w436:T7, "Response"=→"Response":string, "Address Lookup Table Out"=w435:variant)  [unwired: 6 in]
            n158 = Bundle By Name(cluster=w437, "TCP.Refs"=w436, "Addresses.LUT"=w435) -> (w434:T4)
          }
          frame "UI.Disable" {
            n159 = Unbundle By Name(w449) -> ("UI.Refs"=w448:T11)
            n160 = call "Workspace.UI.DisableState.Set.vi"("error in (no error)"=w453, "Enable?"=FALSE, "UI.Refs"=w448) -> ("error out"=w452:errorcluster, "UI.Refs out"=w447:T11)  [unwired: 7 in]
            n161 = Bundle By Name(cluster=w449, "UI.Refs"=w447) -> (w450:T4)
          }
          frame "UI.Enable" {
            n162 = Unbundle By Name(w454) -> ("UI.Refs"=w460:T11)
            n163 = call "Workspace.UI.DisableState.Set.vi"("error in (no error)"=w457, "Enable?"=TRUE, "UI.Refs"=w460) -> ("error out"=w456:errorcluster, "UI.Refs out"=w459:T11)  [unwired: 7 in]
            n164 = Bundle By Name(cluster=w454, "UI.Refs"=w459) -> (w455:T4)
          }
          frame Default {
            n165 = Concatenate Strings(w463, " is not a valid command." ("string")) -> (w462:string)
            n166 = One Button Dialog(message=w462) -> ()  [unwired: 1 in, 1 out]
          }
        }
      }
      frame Error {
        n167 = call <vilib>:"Simple Error Handler.vi"("error in (no error)"=w473) -> ("error out"=w472:errorcluster)  [unwired: 4 in, 4 out]
        n168 = call <vilib>:"Clear Errors.vi"("error in (no error)"=w472) -> ("error out"=w471:errorcluster)  [unwired: 5 in, 1 out]
      }
    }
  }
  n169 = Unbundle By Name(w18) -> ("NIVS.Workspace"=w13:T9, "NIVS.State.Refs"=w14:T10, "State.Notifier"=w16:refnum<user-event>, "LaunchConfig.Ref"=w17:refnum<user-event>, "Events.Refs"=w15:T16, "TCP.Refs"=w12:T7, "Errors.Q"=w11:refnum<queue>)
  n170 = flat-sequence {
    tunnel: w17 -> [w487]
    tunnel: w16 -> [w486]
    tunnel: w15 -> [w485]
    tunnel: w14 -> [w484]
    tunnel: w13 -> [w483]
    tunnel: w12 -> [w477]
    tunnel: w11 -> [w474]
    tunnel: [w482] -> w46
    tunnel: [w481] -> w45
    tunnel: [w480] -> w44
    tunnel: [w479] -> w43
    tunnel: [w478] -> w42
    tunnel: [w476] -> w41
    tunnel: [w475] -> w40
    tunnel: w46 -> [_]
    tunnel: w45 -> [_]
    tunnel: w44 -> [_]
    tunnel: w43 -> [_]
    tunnel: w42 -> [_]
    tunnel: w41 -> [_]
    tunnel: w40 -> [_]
    frame #0 {
      n171 = call <vilib>:"NI VeriStand - Close Workspace Manager Reference.vi"("WorkspaceManager"=w483) -> ("error out"=w482:errorcluster)  [unwired: 10 in]
      n172 = call <vilib>:"NI VeriStand - Close Engine State Change Notification.vi"("SystemStateRefs"=w484) -> ("error out"=w481:errorcluster)  [unwired: 10 in]
      n173 = Destroy User Event(user event=w486) -> (error out=w480:errorcluster)  [unwired: 1 in]
      n174 = Destroy User Event(user event=w487) -> (error out=w479:errorcluster)  [unwired: 1 in]
      n175 = Unregister For Events(event registration refnum=w485) -> (error out=w478:errorcluster)  [unwired: 1 in]
      n176 = call "STM Close Connection.vi"("connection info"=w477) -> ("error out"=w476:errorcluster)  [unwired: 10 in]
      n177 = Release Queue(queue=w474) -> (error out=w475:errorcluster)  [unwired: 2 in, 2 out]
    }
    frame #1 {
    }
  }
